vi "Check Mouse and Snake Face2Face.vi"(8 "error in (no error)":errorcluster, 10 "reference":refnum<class "Snake.lvclass">, 11 "Mouse in":refnum<class "Mouse.lvclass">) -> (0 "error out":errorcluster, 2 "face 2 face?":bool, 3 "Mouse out":refnum<class "Mouse.lvclass">)   [LabVIEW 2021, in "Mouse.lvclass"]
uses:
  Mouse.lvclass
  C:/Users/poche/Programs/LabVIEW/Imposible_Snake/GameEl_class/GameEl.lvclass
  Snake_class/Snake.lvclass
  Mouse.lvclass/Mouse.ctl
  GameEl_class/GameEl.lvclass/GameEl.ctl
  Snake_class/Snake.lvclass/Snake.ctl
  GameEl_class/private/Enum Direction.ctl
  Snake_class/Read Direction.vi
  Snake_class/Read Snake Head.vi
  GameEl_class/Read position.vi
  GameEl_class/GameEl.lvclass
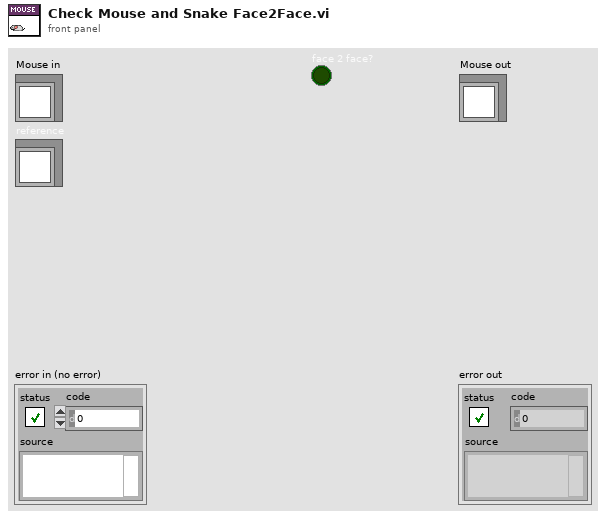
[diagram p1: front panel]
types:
  T1 = typedef "GameEl.lvclass/Enum Direction.ctl" = enum16{"Up", "Down", "Forward", "Backward"}
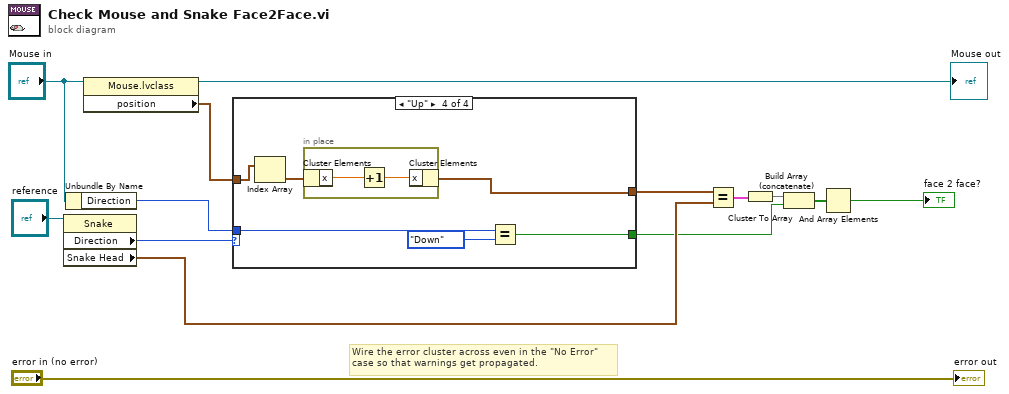
[diagram p0: block diagram]
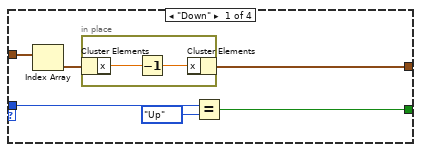
[diagram p2: hidden frame]
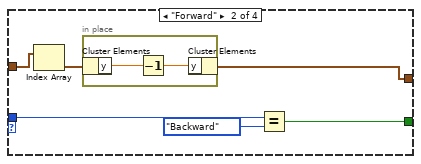
[diagram p3: hidden frame]
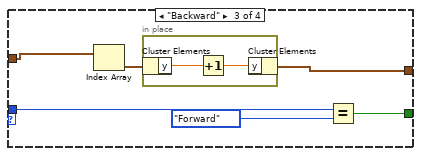
[diagram p4: hidden frame]
diagram:
  # "Wire the error cluster across even in the \"No Error\"\ncase so that warnings get propagated."
  n1 = property class="Snake"(reference="reference") -> ("Direction"=w11:T1, "Snake Head"=w7:cluster{"x":dbl, "y":dbl})  [unwired: 1 in, 2 out]
  n2 = Unbundle By Name("Mouse in") -> ("Direction"=w10:T1)
  n3 = property class="Mouse.lvclass"(reference="Mouse in") -> (reference out=→"Mouse out":refnum<class "Mouse.lvclass">, "position"=w8:cluster{"x":dbl, "y":dbl}[])  [unwired: 1 in, 1 out]
  n4 = case shown="\"Up\"" w11 {
    tunnel: w10 -> [w20 w28 w36 w44]
    tunnel: w8 -> [w18 w25 w33 w41]
    tunnel: [w16 w24 w32 w40] -> w6
    tunnel: [w15 w23 w31 w39] -> w1
    frame "Down" {
      n5 = Index Array(array=w18) -> (element=w17:cluster{"x":dbl, "y":dbl})  [unwired: 1 in]
      n6 = in-place {
        n7 = in-place-cluster #1(w17) -> ("x"=w22:dbl)
        n8 = Decrement(x=w22) -> (x-1=w21:dbl)
        n9 = in-place-cluster #1("x"=w21) -> (w16:cluster{"x":dbl, "y":dbl})
      }
      n10 = Equal?(x=w20, y=Enum_Direction."Up") -> (x = y?=w15:bool)
    }
    frame "Forward" {
      n11 = Index Array(array=w25) -> (element=w26:cluster{"x":dbl, "y":dbl})  [unwired: 1 in]
      n12 = in-place {
        n13 = in-place-cluster #2(w26) -> ("y"=w30:dbl)
        n14 = Decrement(x=w30) -> (x-1=w29:dbl)
        n15 = in-place-cluster #2("y"=w29) -> (w24:cluster{"x":dbl, "y":dbl})
      }
      n16 = Equal?(x=w28, y=Enum_Direction."Backward") -> (x = y?=w23:bool)
    }
    frame "Backward" {
      n17 = Index Array(array=w33) -> (element=w34:cluster{"x":dbl, "y":dbl})  [unwired: 1 in]
      n18 = in-place {
        n19 = in-place-cluster #3(w34) -> ("y"=w38:dbl)
        n20 = Increment(x=w38) -> (x+1=w37:dbl)
        n21 = in-place-cluster #3("y"=w37) -> (w32:cluster{"x":dbl, "y":dbl})
      }
      n22 = Equal?(x=w36, y=Enum_Direction."Forward") -> (x = y?=w31:bool)
    }
    frame "Up" {
      n23 = Index Array(array=w41) -> (element=w42:cluster{"x":dbl, "y":dbl})  [unwired: 1 in]
      n24 = in-place {
        n25 = in-place-cluster #4(w42) -> ("x"=w46:dbl)
        n26 = Increment(x=w46) -> (x+1=w45:dbl)
        n27 = in-place-cluster #4("x"=w45) -> (w40:cluster{"x":dbl, "y":dbl})
      }
      n28 = Equal?(x=w44, y=Enum_Direction."Down") -> (x = y?=w39:bool)
    }
  }
  n29 = Equal?(x=w6, y=w7) -> (x = y?=w5:cluster{"x":bool, "y":bool})
  n30 = Cluster To Array(cluster=w5) -> (array=w4:bool[])
  n31 = Build Array (concatenate)(w4, w1) -> (w2:bool[])
  n32 = And Array Elements(Boolean array=w2) -> (logical AND=→"face 2 face?":bool)
  "error out" <- "error in (no error)"
